vi "Configure Payload Frames RTM.vi"(8 "error in (no error)":errorcluster, 11 "Node Ptr":u64 format="%.0x") -> (0 "error out":errorcluster)   [LabVIEW 2020, in "AIM ARINC 664 System Explorer.lvlib" / "Implementation.lvlib"]
uses:
  Implementation.lvlib
  Scripting/AIM ARINC 664 Scripting.lvlib
  <vilib>/Utility/SystemLogging/NI_SystemLogging.lvlib
  <vilib>/NI VeriStand/Custom Device Tools/Custom Device Utility Library/Custom Device Utility Library.lvlib
  <vilib>/NI VeriStand/Custom Device API/Custom Device API.lvlib
  Frame Configuration/FrameEditor.lvlib
panel:
  in  "Tag":string
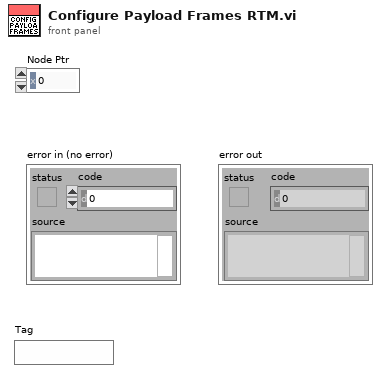
[diagram p1: front panel]
types:
  T1 = typedef "Custom Device API.lvlib/Custom Device Item Ref.ctl" = u64
  T2 = typedef "Payload Map.ctl" = map{string, T3}
  T3 = typedef "Payload Record Type.ctl" = cluster{"Data":u8[], "Type of Frame":T4}
  T4 = typedef "Type of Payload.ctl" = u16
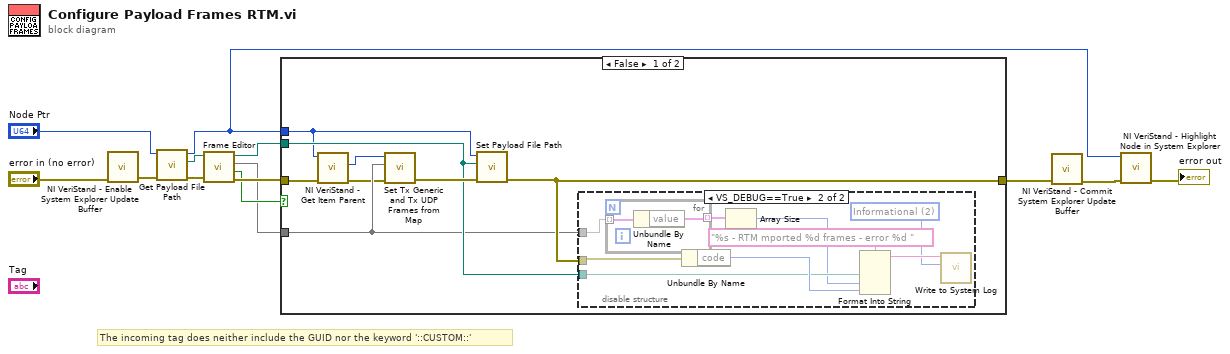
[diagram p0: block diagram]
diagram:
  # "The incoming tag does neither include the GUID nor the keyword '::CUSTOM::'"
  n1 = call <vilib>:"NI VeriStand - Enable System Explorer Update Buffer.vi"("error in (no error)"="error in (no error)") -> ("error out"=w5:errorcluster)  [unwired: 10 in]
  n2 = call "Get Payload File Path.vi"("error in"=w5, "custom device ref in"="Node Ptr") -> ("error out"=w3:errorcluster, "frame array file path"=w2:path, "custom device ref out"=w1:T1)  [unwired: 4 in, 3 out]
  n3 = call "Frame Editor.vi"("error in"=w3, "Input File"=w2) -> ("error out"=w13:errorcluster, "Cancelled"=w12:bool, "Output Map"=w11:T2, "Currently Loaded file"=w10:path)  [unwired: 6 in]
  n4 = case shown="False" w12 {
    tunnel: w13 -> [w17 w33]
    tunnel: [w20 w33] -> w8
    tunnel: w1 -> [w15 _]
    tunnel: w11 -> [w18 _]
    tunnel: w10 -> [w19 _]
    frame False {
      n5 = call <vilib>:"NI VeriStand - Get Item Parent.vi"("error in (no error)"=w17, "Item Ref in"=w15) -> ("error out"=w16:errorcluster, "Parent Ref"=w14:T1)  [unwired: 6 in, 2 out]
      n6 = call "Set Tx Generic and Tx UDP Frames from Map.vi"("error in"=w16, "payload map"=w18, "custom device ref"=w14) -> ("error out"=w21:errorcluster)  [unwired: 7 in, 1 out]
      n7 = call "Set Payload File Path.vi"("error in"=w21, "frame array file path"=w19, "custom device ref in"=w15) -> ("error out"=w20:errorcluster)  [unwired: 7 in, 1 out]
      n8 = disable-structure shown="VS_DEBUG==True" {
        disable-tunnel: w20 -> [_ w27]
        disable-tunnel: w19 -> [_ w25]
        disable-tunnel: w18 -> [_ w23]
        frame condition #0 (active) {
        }
        frame condition #1 {
          w28 = 2 items=["Error", "Warning", "Informational"] ("severity")
          n9 = for {
            tunnel: w23 -> [w32] mode=indexing
            tunnel: [w31] -> w22 mode=indexing
            n10 = Unbundle By Name(w32) -> ("value"=w31:T3)
          }
          n11 = Unbundle By Name(w27) -> ("code"=w26:i32)
          n12 = Array Size(array=w22) -> (size(s)=w24:i32)
          n13 = Format Into String(format string="%s - RTM mported %d frames - error %d ", w25, w24, w26) -> (resulting string=w29:string)  [unwired: 2 in, 1 out]
          n14 = call <vilib>:"Write to System Log.vi"("severity"=w28, "message"=w29) -> ()  [unwired: 9 in, 1 out]
        }
      }
    }
    frame True {
    }
  }
  n15 = call <vilib>:"NI VeriStand - Commit System Explorer Update Buffer.vi"("error in (no error)"=w8) -> ("error out"=w7:errorcluster)  [unwired: 10 in]
  n16 = call <vilib>:"NI VeriStand - Highlight Node in System Explorer.vi"("error in (no error)"=w7, "Item Ref in"=w1) -> ("error out"=→"error out":errorcluster)  [unwired: 8 in, 1 out]
